vi "Main.vi"() -> ()   [LabVIEW 2024]
uses:
  Support/Type Defs/QMH Message--cluster.ctl
  <vilib>/Utility/miscctls.llb/LVRectTypeDef.ctl
  Pages/Timer Page.vi
  View.lvlib
panel:
  in  "Stop":bool
  in  "Settings Button":bool
  in  "Start Button":bool
  # "Locals"
  # "Made by Ramazan Burak Korkmaz 2025"
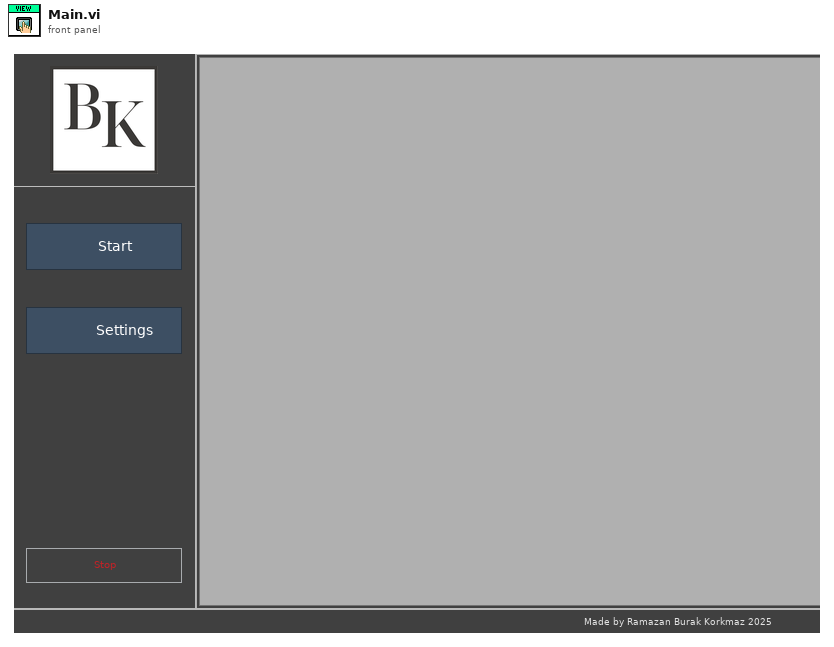
[diagram p1: front panel]
types:
  T1 = typedef "View.lvlib/QMH Message--cluster.ctl" = cluster{"Message":string, "Message Data":variant}
  T2 = typedef "LVRectTypeDef.ctl" = cluster{"Left":i16, "Top":i16, "Right":i16, "Bottom":i16}
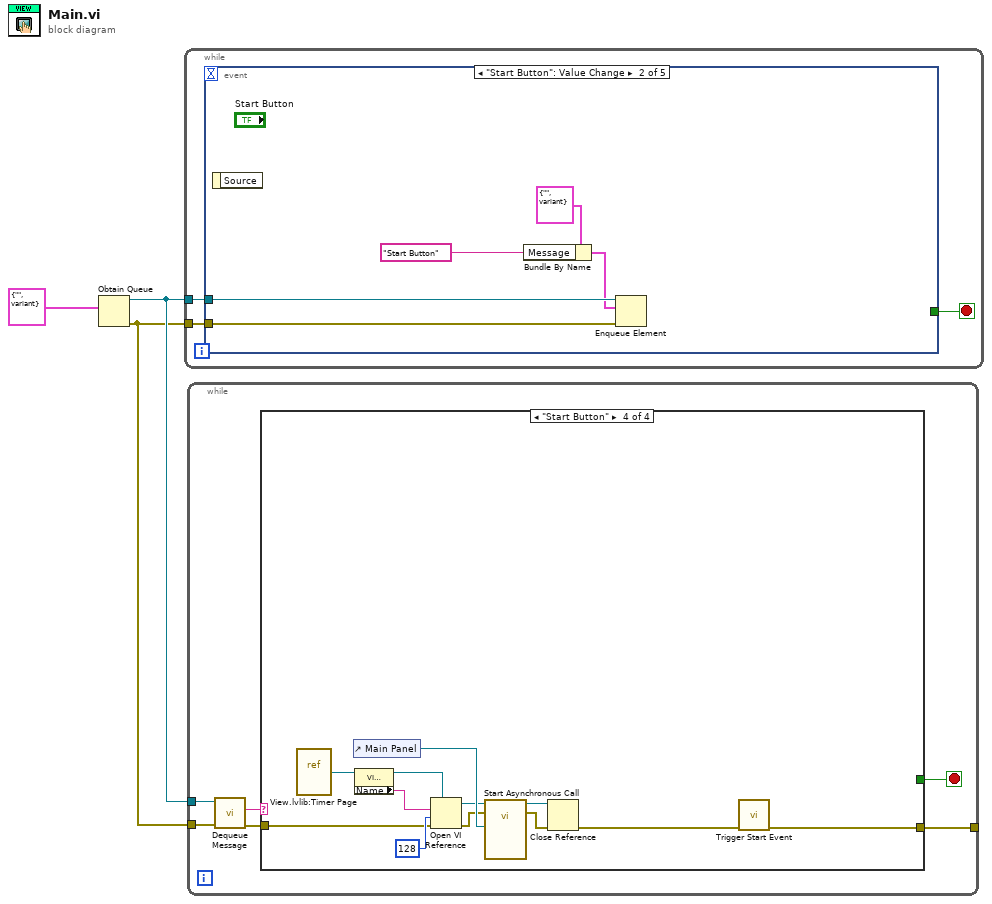
[diagram p0: block diagram]
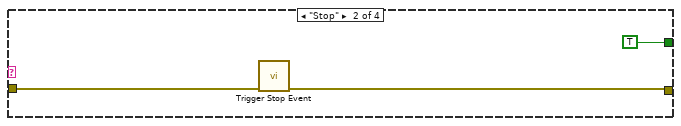
[diagram p3: hidden frame]
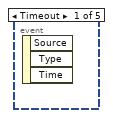
[diagram p5: hidden frame]
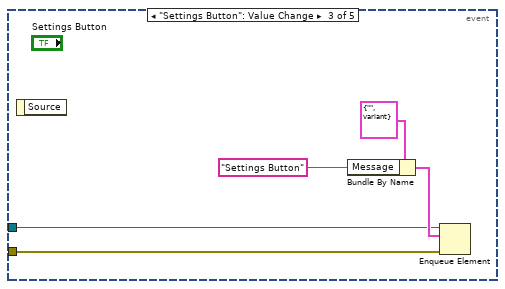
[diagram p6: hidden frame]
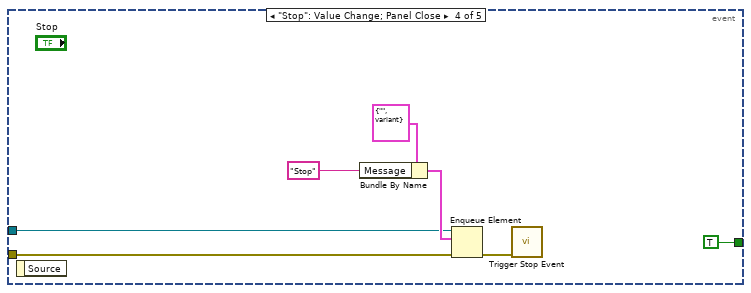
[diagram p7: hidden frame]
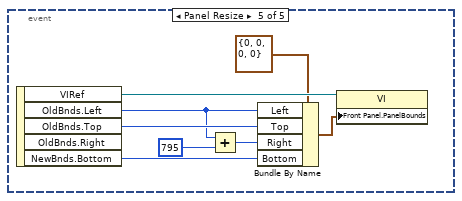
[diagram p8: hidden frame]
diagram:
  n1 = Obtain Queue(element data type=T1 {"Message"="", "Message Data"=variant} ("Message")) -> (queue out=w2:refnum<queue>, error out=w1:errorcluster)  [unwired: 4 in, 1 out]
  n2 = while {
    tunnel: w2 -> [w6]
    tunnel: w1 -> [w5]
    stop <- w4 stop-if-true
    n3 = event shown="[1] \"Start Button\": Value Change" {
      selector: _ -> [_ _ _ _ _]
      dyn-events: _ -> [_ _ _ _ _]
      timeout: _ -> [_ _ _ _ _]
      tunnel: w6 -> [_ w11 w14 w20 _]
      tunnel: w5 -> [_ w10 w13 w18 _]
      tunnel: [_ _ _ TRUE _] -> w4
      event Timeout {
        n4 = event-data() -> ()  [unwired: 1 in, 3 out]
      }
      event "Start Button": Value Change {
        n5 = event-data() -> ()  [unwired: 1 in, 1 out]
        n6 = Bundle By Name(cluster=T1 {"Message"="", "Message Data"=variant} ("element"), "Message"="Start Button") -> (w8:T1)
        n7 = Enqueue Element(queue=w11, element=w8, error in (no error)=w10) -> ()  [unwired: 1 in, 3 out]
      }
      event "Settings Button": Value Change {
        n8 = event-data() -> ()  [unwired: 1 in, 1 out]
        n9 = Bundle By Name(cluster=T1 {"Message"="", "Message Data"=variant} ("element"), "Message"="Settings Button") -> (w15:T1)
        n10 = Enqueue Element(queue=w14, element=w15, error in (no error)=w13) -> ()  [unwired: 1 in, 3 out]
      }
      event "Stop": Value Change; Panel Close {
        n11 = event-data() -> ()  [unwired: 1 in, 1 out]
        n12 = Bundle By Name(cluster=T1 {"Message"="", "Message Data"=variant} ("element"), "Message"="Stop") -> (w22:T1)
        n13 = Enqueue Element(queue=w20, element=w22, error in (no error)=w18) -> (error out=w17:errorcluster)  [unwired: 1 in, 2 out]
        n14 = call "Trigger Stop Event.vi"("error in (no error)"=w17) -> ()  [unwired: 10 in, 1 out]
      }
      event Panel Resize {
        n15 = event-data() -> ("VIRef"=w31:refnum<vi>, "OldBnds.Left"=w24:i16, "OldBnds.Top"=w28:i16, "NewBnds.Bottom"=w27:i16)  [unwired: 1 in, 1 out]
        n16 = Add(x=w24, y=i16 795 ("Right")) -> (x+y=w25:i16)
        n17 = Bundle By Name(cluster=T2 {"Left"=0, "Top"=0, "Right"=0, "Bottom"=0} ("Front Panel Window:Panel Bounds"), "Left"=w24, "Top"=w28, "Right"=w25, "Bottom"=w27) -> (w29:T2)
        n18 = property class="VI"(reference=w31, "Front Panel.PanelBounds"=w29) -> ()  [unwired: 1 in, 2 out]
      }
    }
  }
  n19 = while {
    tunnel: w2 -> [w37]
    tunnel: w1 -> [w36]
    tunnel: [w33] -> _
    stop <- w32 stop-if-true
    n20 = call "Dequeue Message.vi"("error in (no error)"=w36, "Queue in"=w37) -> ("error out"=w34:errorcluster, "Message"=w35:string)  [unwired: 7 in, 1 out]
    n21 = case shown="\"Start Button\"" w35 {
      tunnel: w34 -> [w38 w40 w42 w45]
      tunnel: [w38 w39 w42 w43] -> w33
      tunnel: [_ TRUE _ _] -> w32
      frame "Settings Button" {
      }
      frame "Stop" {
        n22 = call "Trigger Stop Event.vi"("error in (no error)"=w40) -> ("error out"=w39:errorcluster)  [unwired: 10 in]
      }
      frame Default {
      }
      frame "Start Button" {
        n23 = vi-ref "View.lvlib:Timer Page.vi"() -> (w49:refnum<vi>)
        n24 = control-ref of="Main Panel"() -> (w54:refnum<vi>)
        n25 = property class="VI (strict)"(reference=w49) -> (reference out=w50:refnum<vi>, "Name"=w51:string)  [unwired: 1 in, 1 out]
        n26 = Open VI Reference(type specifier VI Refnum (for type only)=w50, vi path=w51, options=128, error in (no error)=w45) -> (vi reference=w47:refnum<vi>, error out=w48:errorcluster)  [unwired: 2 in]
        n27 = call-by-ref "Start Asynchronous Call"(reference=w47, error in=w48, "Main Panel"=w54) -> (reference out=w52:refnum<vi>, error out=w53:errorcluster)  [unwired: 11 in]
        n28 = Close Reference(reference=w52, error in (no error)=w53) -> (error out=w44:errorcluster)
        n29 = call "Trigger Start Event.vi"("error in (no error)"=w44) -> ("error out"=w43:errorcluster)  [unwired: 10 in]
      }
    }
  }
